vi "DAQmx Rolling Average.vi"(5 "Sample Rate":dbl=100.0, 7 "Seconds to Average":dbl=100.0, 8 "Signal":dynamicdata(waveform), 9 "Action":enum16{"Average", "Init"}(ring)=enum."Init", 11 "Sample Size":i32=100) -> (3 "Mean Array":dbl[](array[numeric]))   [LabVIEW 2018]
uses:
  <vilib>/Analysis/baseanly.llb/Mean (DBL).vi
  <vilib>/Analysis/NI_AALBase.lvlib
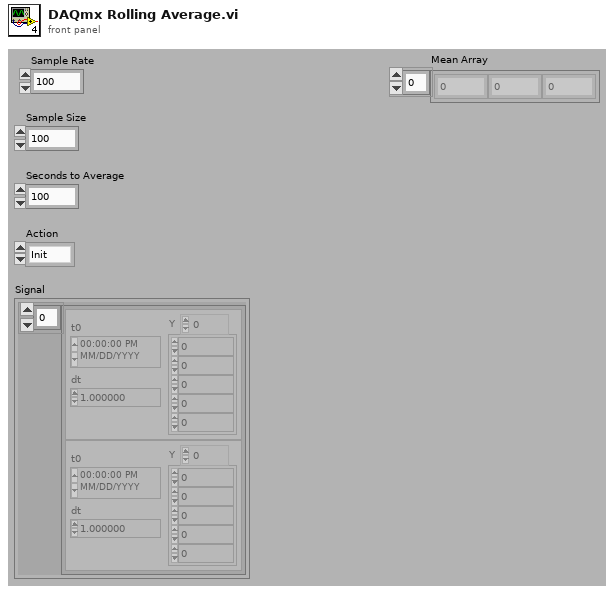
[diagram p1: front panel]
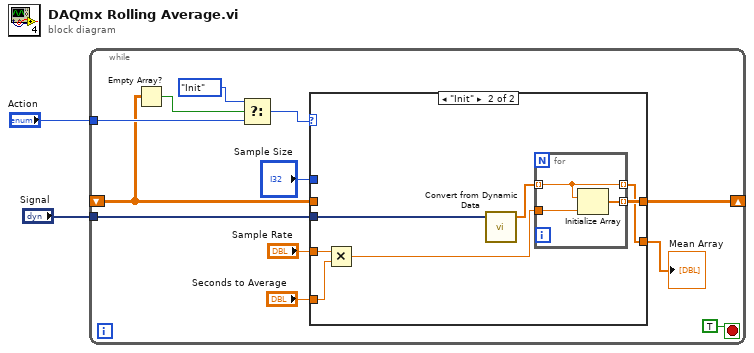
[diagram p0: block diagram]
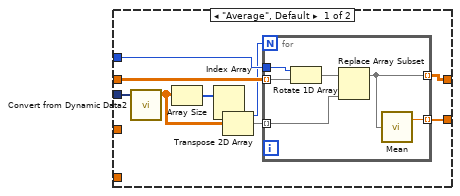
[diagram p2: hidden frame]
diagram:
  n1 = while {
    shift-right: [w13] -> _
    shift-left: _ -> [w5]
    tunnel: "Signal" -> [w8]
    tunnel: "Action" -> [w7]
    stop <- TRUE stop-if-true
    n2 = Empty Array?(array=w5) -> (empty?=w4:bool)
    n3 = Select(t=enum16{"Average", "Init"}."Init", s=w4, f=w7) -> (s? t:f=w6:enum16{"Average", "Init"})
    n4 = case shown="\"Init\"" w6 {
      tunnel: w5 -> [w23 _]
      tunnel: "Sample Size" -> [w19 _]
      tunnel: [w20 w31] -> w9
      tunnel: [w21 w32] -> w13
      tunnel: "Seconds to Average" -> [_ w36]
      tunnel: "Sample Rate" -> [_ w35]
      tunnel: w8 -> [w22 w34]
      frame "Average", Default {
        n5 = call "Convert from Dynamic Data2"("Dynamic Data Type"=w22) -> ("Array"=w18:dbl[][])  [unwired: 3 in]
        n6 = Array Size(array=w18) -> (size(s)=w17:i32[])
        n7 = Index Array(array=w17) -> (element #2=w16:i32)  [unwired: 2 in, 1 out]
        n8 = Transpose 2D Array(2D array=w18) -> (transposed array=w15:dbl[][])
        n9 = for {
          N: w16 -> [_]
          tunnel: w23 -> [w29] mode=indexing
          tunnel: w15 -> [w27] mode=indexing
          tunnel: [w26] -> w21 mode=indexing
          tunnel: [w25] -> w20 mode=indexing
          tunnel: w19 -> [w24]
          n10 = Rotate 1D Array(1:w29, 2:w24) -> (0:w28:dbl[])
          n11 = Replace Array Subset(array=w28, new element=w27) -> (w26:dbl[])  [unwired: 1 in]
          n12 = call-poly <vilib>:"Mean.vi"("X"=w26) -> ("mean"=w25:dbl)  [unwired: 1 out]
        }
      }
      frame "Init" {
        n13 = Multiply(x=w35, y=w36) -> (x*y=w33:dbl)
        n14 = call "Convert from Dynamic Data"("Dynamic Data Type"=w34) -> ("Array"=w30:dbl[])  [unwired: 3 in]
        n15 = for {
          tunnel: w30 -> [w37] mode=indexing
          tunnel: w33 -> [w39]
          tunnel: [w38] -> w32 mode=indexing
          tunnel: [w37] -> w31 mode=indexing
          n16 = Initialize Array(w37, w39) -> (w38:dbl[])
        }
      }
    }
    "Mean Array" <- w9
  }
